vi "Eye_Recorder_v1.0.vi"() -> ()   [LabVIEW 2019]
uses:
  <vilib>/vision/driver/IMAQdx.llb/IMAQdx Acquisition Mode.ctl
  <vilib>/vision/driver/IMAQdx.llb/IMAQdx Buffer Number Mode.ctl
  <vilib>/MakerHub/LINX/Public/Peripherals/Analog/Analog Read N Chans.vi
  <vilib>/MakerHub/LINX/Private/Local IO/LinxAnalogRead.vi
  <vilib>/MakerHub/LINX/Public/Utilities/Check Channel.vi
  <vilib>/MakerHub/LINX/Public/Utilities/Open Serial.vi
  <vilib>/MakerHub/LINX/Private/Utilties/Generate Error.vi
  <vilib>/Utility/file.llb/Write Delimited Spreadsheet (DBL).vi
  <vilib>/vision/driver/NI_Vision_Acquisition_Software.lvlib
  <resource>/objmgr/imaqdx.rc
  <vilib>/vision/NI_Vision_Development_Module.lvlib
  <vilib>/MakerHub/LINX/LMH-LINX.lvlib
panel:
  out "Recording Status":i16[](graph)
  out "Button Status":i16[](graph)
  in  "AI Channel(s)":u8[](array[numeric])=[0, 1]
  out "Experiment Status":i16[](graph)
  in  "AI Threshold":dbl=2.0
  in  "Serial Port":refnum<visa-resource-name>="COM9"
  out "Data Valid":bool
  in  "Centroid Distance Threshold":sgl=5.0
  in  "Initial SD Threshold":sgl=4.0
  in  "SD Threshold Ratio for Stop":sgl=1.2
  in  "SD Threshold Ratio for Start":sgl=1.5
  out "Writing":bool
  in  "Number of Buffered Frames":i32=200
  in  "Smart Record Enable":bool
  out "Actual Frame Rate":dbl=50.04906771344455
  out "Missed Frames":bool
  out "Standard Variation":sgl=5.0659676
  out "Centroid":cluster{"X Centroid":sgl, "Y Centroid":sgl}={"X Centroid"=323.0136, "Y Centroid"=231.01224} {"Y Centroid" format="%.2f"; "X Centroid" format="%.2f"}
  out "Manual ROI":T1={"Global Rectangle"=[0, 0, 639, 479], "Contours"=[{"Contour Type"=0, "ROI Type"=12, "Points"=[0, 0, 639, 479, 0]}]}
  in  "Image Type":T2 items=["Grayscale (U8)", "Grayscale (I16)", "Grayscale (SGL)", "Complex (CSG)", "RGB (U32)", "HSL (U32)", "RGB (U64)", "Grayscale (U16)"]
  in  "Camera Type":enum16{"Basler", "Mako"}(ring)=enum."Mako"
  in  "Folder Path":path=path "C:/Users/VR1/Documents/EyeTrackin/Diego_103019"
  in  "Exposure Time (us)":dbl=15000.0
  out "error out":errorcluster
  in  "Stop":bool
  in  "Byte Order":T3(ring)=enum."little-endian"
  in  "Record?":bool
  in  "File Name (.mtif)":string="test_1"
  out "Size":cluster{"X":i32, "Y":i32}={"X"=640, "Y"=480}
  out "Actual Camera ROI":T4={"Left"=0, "Top"=0, "Right"=639, "Bottom"=479, "Rotation"=0.0} {"Rotation" format="%.2f"; "Left" scale=0.0..1024.0; "Right" scale=0.0..1024.0}
  in  "Set Camera ROI":T4={"Left"=0, "Top"=0, "Right"=639, "Bottom"=479, "Rotation"=0.0} {"Rotation" min=-90.0 max=90.0 step=1.0 format="%.2f"; "Left" scale=0.0..1024.0; "Right" scale=0.0..1024.0}
  out "Raw Image":T5(plugin-control)
  in  "Frame Rate (fps)":dbl=50.0
  in  "Camera Name":refnum<k21>="cam0" caption="IMAQdx Session"
  in  "error in":errorcluster
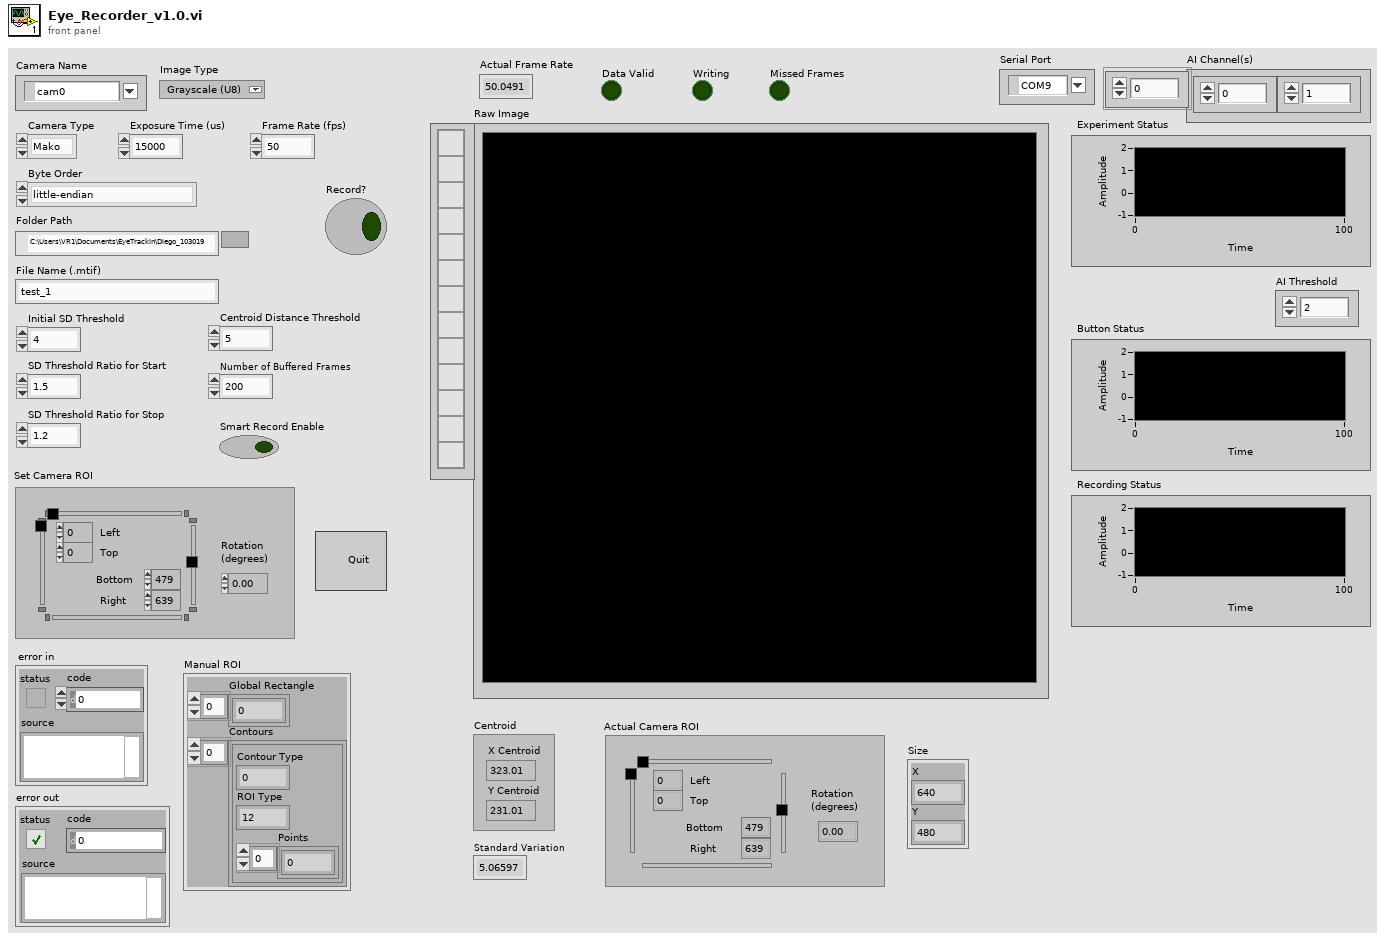
[diagram p1: front panel]
types:
  T1 = cluster{"Global Rectangle":i32[], "Contours":cluster{"Contour Type":u32, "ROI Type":u32, "Points":i32[]}[]}
  T2 = typedef "Image Type" = u32
  T3 = enum16{"big-endian, network order", "native, host order", "little-endian"}
  T4 = typedef "IMAQ Rectangle" = cluster{"Left":i32, "Top":i32, "Right":i32, "Bottom":i32, "Rotation":dbl}
  T5 = typedef "IMAQ Image.ctl" = refnum<image>
  T6 = cluster{"Standard Variation":sgl, "Centroid":cluster{"X Centroid":sgl, "Y Centroid":sgl}}
  T7 = cluster{"ImgDataArray":u8[], "Standard Variation":sgl, "Centroid":cluster{"X Centroid":sgl, "Y Centroid":sgl}}
  T8 = typedef "NI_Vision_Acquisition_Software.lvlib/IMAQdx Acquisition Mode.ctl" = enum32{"One Shot", "Continuous"}
  T9 = typedef "IMAQdx.ctl" = refnum<k21>
  T10 = cluster{"Global Rectangle":i32[], "Contours":cluster{"Contour Type":u32, "Type":u32, "Coordinates":i32[]}[]}
  T11 = typedef "LMH-LINX.lvlib/LINX Ref.ctl" = cluster{"IO":T12, "Interface":T13, "LINX Device Config":T14}
  T12 = typedef "LMH-LINX.lvlib/Platform.ctl" = enum16{"Remote", "Local"}
  T13 = typedef "LMH-LINX.lvlib/Interface.ctl" = enum16{"Serial", "TCP"}
  T14 = typedef "LMH-LINX.lvlib/Device.lvlib/LINX Device Config.ctl" = cluster{"Interface":T13, "COM Port":refnum<visa-resource-name>, "TCP Configuration":T15, "Device Family":u8, "Device ID":u8, "Device Name":string, "TCP Ref":refnum<k5>, "Channels":T16}
  T15 = typedef "LMH-LINX.lvlib/Device.lvlib/TCP Config.ctl" = cluster{"IP Address":string, "Port":u16}
  T16 = typedef "LMH-LINX.lvlib/Channels.ctl" = cluster{"DI":u8[], "DO":u8[], "AI":u8[], "AO":u8[], "PWM":u8[], "QE":u8[], "UART":u8[], "I2C 2":u8[], "SPI":u8[], "CAN":u8[], "Servo":u8[], "AI Ref (V)":dbl, "AI Resolution (Bits)":u8, "AO Ref (V)":dbl, "AO Resolution (Bits)":u8}
  T17 = typedef "NI_Vision_Acquisition_Software.lvlib/IMAQdx Buffer Number Mode.ctl" = enum32{"Next", "Last", "Buffer Number", "Every", "Last New"}
  T18 = cluster{"Mean Value":sgl, "Standard Variation":sgl, "Minimal Value":sgl, "Maximal Value":sgl, "Area (calibrated)":sgl, "Area (pixels)":u32, "%":sgl, "Calibration Valid":bool}
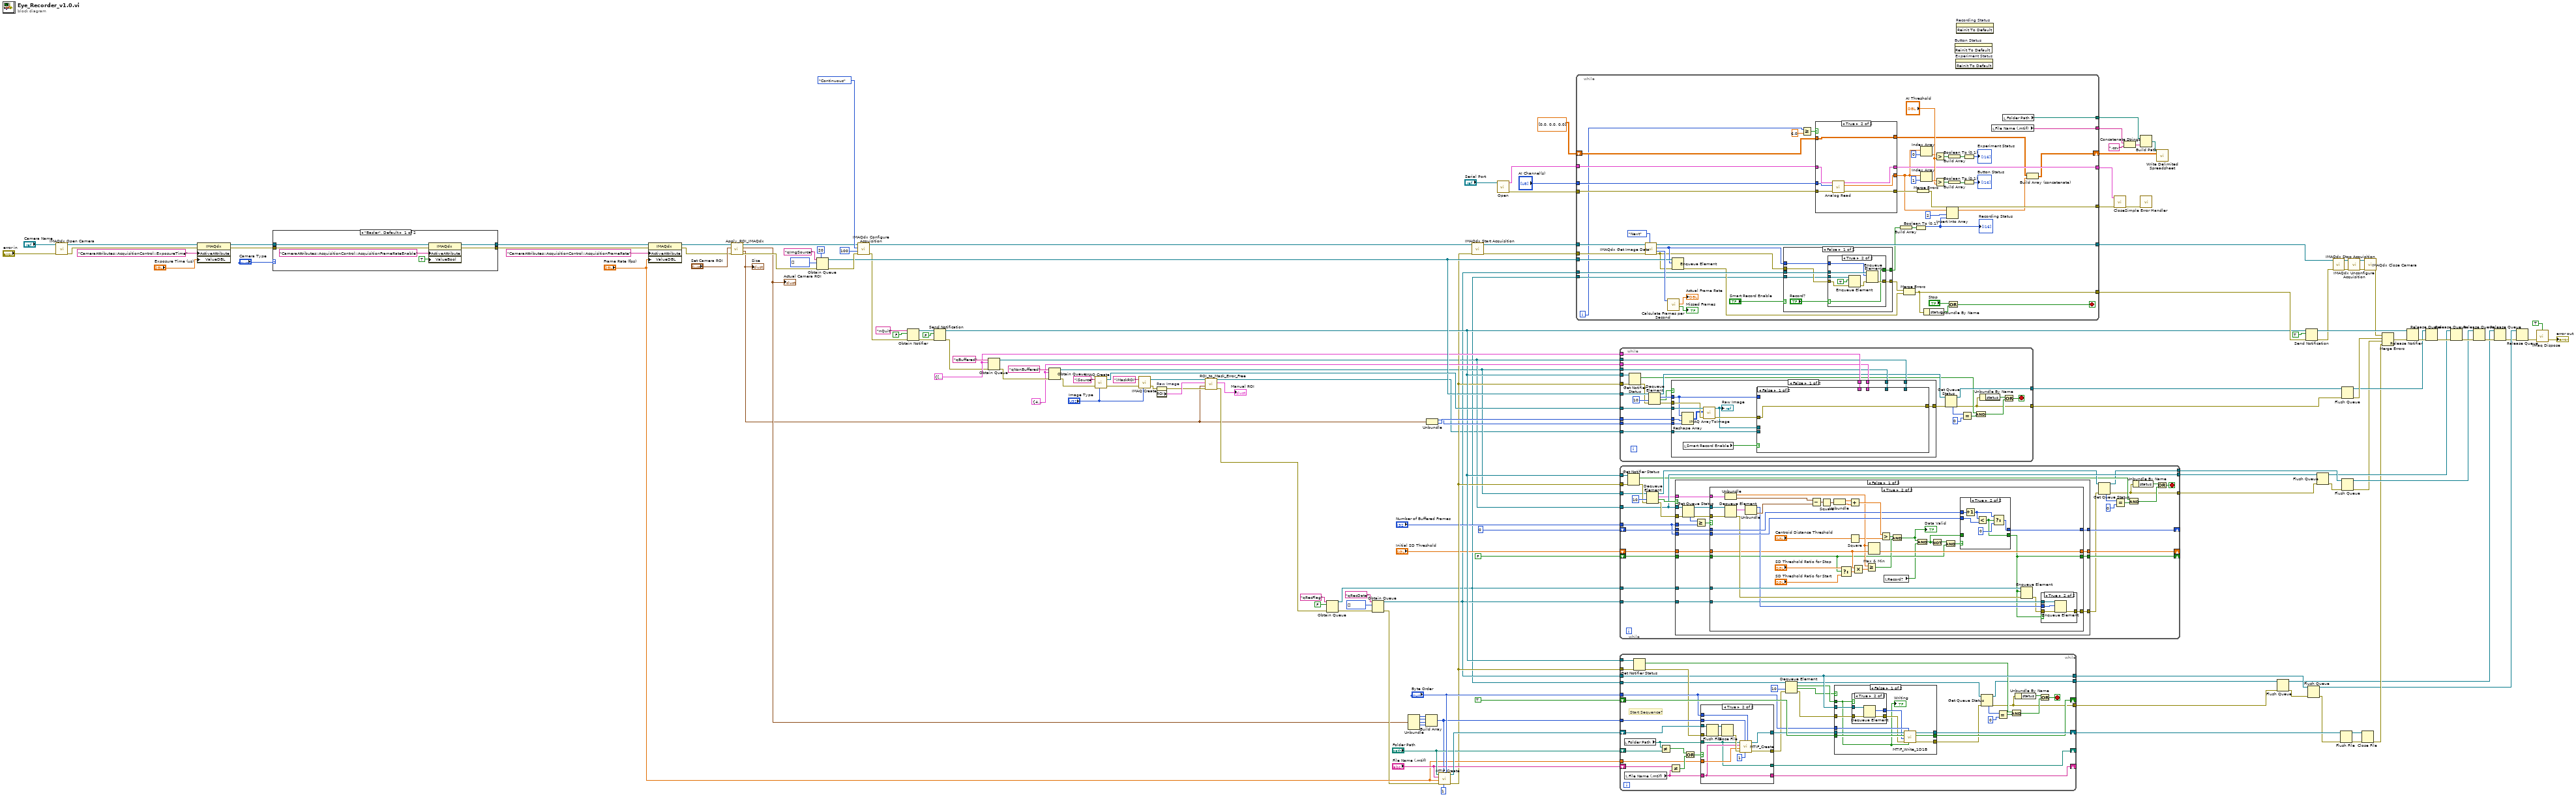
[diagram p0: block diagram]
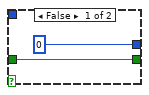
[diagram p4: hidden frame]
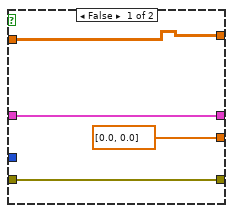
[diagram p6: hidden frame]
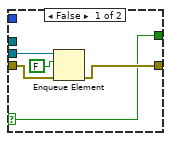
[diagram p7: hidden frame]
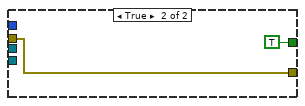
[diagram p8: hidden frame]
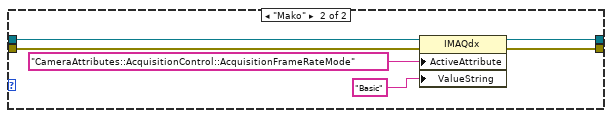
[diagram p9: hidden frame]
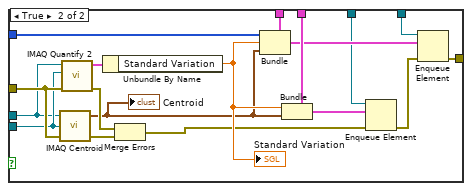
[diagram p10: hidden frame]
diagram:
  w66 = T6 {"Standard Variation"=4836.523, "Centroid"={"X Centroid"=313.66412, "Y Centroid"=260.78278}}
  w67 = T7 {"ImgDataArray"=[], "Standard Variation"=4836.523, "Centroid"={"X Centroid"=313.66412, "Y Centroid"=260.78278}}
  n1 = call <vilib>:"IMAQdx Open Camera.vi"("error in"="error in", "Session In"="Camera Name") -> ("error out"=w96:errorcluster, "Session Out"=w97:T9)  [unwired: 1 in, 7 out]
  n2 = property class="IMAQdx"(reference=w97, error in=w96, "ActiveAttribute"="CameraAttributes::AcquisitionControl::ExposureTime", "ValueDBL"="Exposure Time (us)") -> (reference out=w95:T9, error out=w94:errorcluster)
  n3 = case shown="\"Basler\", Default" "Camera Type" {
    tunnel: w95 -> [w145 w151]
    tunnel: w94 -> [w144 w150]
    tunnel: [w143 w149] -> w93
    tunnel: [w142 w148] -> w92
    frame "Basler", Default {
      n4 = property class="IMAQdx"(reference=w145, error in=w144, "ActiveAttribute"="CameraAttributes::AcquisitionControl::AcquisitionFrameRateEnable", "ValueBool"=TRUE) -> (reference out=w143:T9, error out=w142:errorcluster)
    }
    frame "Mako" {
      n5 = property class="IMAQdx"(reference=w151, error in=w150, "ActiveAttribute"="CameraAttributes::AcquisitionControl::AcquisitionFrameRateMode", "ValueString"="Basic") -> (reference out=w149:T9, error out=w148:errorcluster)
    }
  }
  n6 = property class="IMAQdx"(reference=w93, error in=w92, "ActiveAttribute"="CameraAttributes::AcquisitionControl::AcquisitionFrameRate", "ValueDBL"="Frame Rate (fps)") -> (reference out=w91:T9, error out=w90:errorcluster)
  n7 = call "Apply_ROI_IMAQdx.vi"("error in (no error)"=w90, "ROI"="Set Camera ROI", "Session in"=w91) -> ("error out"=w116:errorcluster, "Size"=w15:cluster{"X":i32, "Y":i32}, "Actual ROI"=w16:T4, "Session out"=w134:T9)  [unwired: 5 in]
  "Actual Camera ROI" <- w16
  "Size" <- w15
  n8 = Obtain Queue(max queue size (-1, unlimited)=20, name (unnamed)="qImgSource", element data type=u8[] [] ("Image Data Array"), error in (no error)=w116) -> (queue out=w76:refnum<queue>, error out=w115:errorcluster)  [unwired: 1 in, 1 out]
  n9 = call <vilib>:"IMAQdx Configure Acquisition.vi"("error in"=w115, "Number of Buffers"=u32 100, "Continuous?"=IMAQdx_Acquisition_Mode."Continuous", "Session In"=w134) -> ("error out"=w64:errorcluster, "Session Out"=w121:T9)  [unwired: 6 in]
  n10 = Obtain Notifier(name (unnamed)="nQuit", notification data type=FALSE ("element"), error in (no error)=w64) -> (notifier out=w111:refnum<notifier>, error out=w110:errorcluster)  [unwired: 1 in, 1 out]
  n11 = Send Notification(notification=FALSE, notifier=w111, error in (no error)=w110) -> (notifier out=w60:refnum<notifier>, error out=w63:errorcluster)
  n12 = Obtain Queue(name (unnamed)="qBuffered", element data type=w67, error in (no error)=w63) -> (queue out=w58:refnum<queue>, error out=w70:errorcluster)  [unwired: 2 in, 1 out]
  n13 = Obtain Queue(name (unnamed)="qNonBuffered", element data type=w66, error in (no error)=w70) -> (queue out=w57:refnum<queue>, error out=w68:errorcluster)  [unwired: 2 in, 1 out]
  n14 = call "IMAQ Create"("Image Name"="iSource", "Image Type"="Image Type", "error in (no error)"=w68) -> ("New Image"=w80:T5, "error out"=w81:errorcluster)  [unwired: 2 in]
  n15 = call "IMAQ Create"("Image Name"="iMaskROI", "Image Type"="Image Type", "error in (no error)"=w81) -> ("New Image"=w22:T5, "error out"=w25:errorcluster)  [unwired: 2 in]
  n16 = property on="Raw Image" class="ImageControl"(error in=w25) -> (error out=w20:errorcluster, "ROI"=w21:T1)  [unwired: 1 in, 1 out]
  n17 = call "ROI_to_Mask_Error_Free.vi"("error in (no error)"=w20, "Image Size"=w15, "ROI in"=w21, "Refnum in"=w22) -> ("error out"=w17:errorcluster, "ROI out"=→"Manual ROI":T10, "Refnum out"=w19:T5)  [unwired: 5 in]
  n18 = Obtain Queue(name (unnamed)="qRecFlag", element data type=FALSE, error in (no error)=w17) -> (queue out=w23:refnum<queue>, error out=w41:errorcluster)  [unwired: 2 in, 1 out]
  n19 = Obtain Queue(name (unnamed)="qRecData", element data type=u8[] [] ("Image Data Array"), error in (no error)=w41) -> (queue out=w24:refnum<queue>, error out=w38:errorcluster)  [unwired: 2 in, 1 out]
  n20 = Unbundle(w16) -> ("Left"=w133:i32, "Top"=w132:i32, "Right"=w131:i32, "Bottom"=w130:i32)  [unwired: 1 out]
  n21 = Build Array(w133, w132, w131, w130) -> (w84:i32[])
  n22 = Unbundle(w15) -> ("X"=w103:i32, "Y"=w104:i32)
  n23 = call "MTIF_Create.vi"("Byte Order"="Byte Order", "Bytes per pixel"=u8 1, "ROI Rectangle"=w84, "error in (no error)"=w38, "Frame Rate (fps)"="Frame Rate (fps)", "File Name (.mtif)"="File Name (.mtif)", "Folder Path"="Folder Path") -> ("error out"=w59:errorcluster, "Byte Stream File out"=w129:refnum<file>)  [unwired: 3 in]
  n24 = call <vilib>:"IMAQdx Start Acquisition.vi"("error in"=w59, "Session In"=w121) -> ("error out"=w77:errorcluster, "Session Out"=w78:T9)  [unwired: 8 in]
  n25 = call-poly <vilib>:"Open.vi"("Serial Port"="Serial Port") -> ("Error Out"=w3:errorcluster, "LINX Resource"=w2:T11)  [unwired: 8 in, 1 out]
  n26 = while {
    tunnel: w78 -> [w200]
    tunnel: w77 -> [w199]
    tunnel: [w196] -> w74
    tunnel: w76 -> [w193]
    tunnel: [w187] -> w73
    tunnel: w24 -> [w190]
    tunnel: w23 -> [w183]
    tunnel: [w168] -> w11
    tunnel: [w167] -> w9
    tunnel: [w166] -> w8
    tunnel: [w165] -> w7
    tunnel: "AI Channel(s)" -> [w164]
    tunnel: w3 -> [w162]
    tunnel: w2 -> [w161]
    shift-right: [w152] -> w1
    shift-left: dbl[][] [[0.0, 0.0, 0.0]] -> [w163]
    i -> [w160]
    stop <- w195 stop-if-true
    n27 = call <vilib>:"IMAQdx Get Image Data.vi"("Buffer Number Mode (Next)"=IMAQdx_Buffer_Number_Mode."Next", "error in"=w199, "Session In"=w200) -> ("error out"=w188:errorcluster, "Buffer Number Out"=w197:u32, "Image Data Array"=w189:u8[], "Session Out"=w196:T9)  [unwired: 5 in]
    n28 = call <vilib>:"Calculate Frames per Second.vi"("Buffer Number"=w197) -> ("Missed Frames"=→"Missed Frames":bool, "Processed Frames/s"=→"Actual Frame Rate":dbl)  [unwired: 8 in, 1 out]
    n29 = Enqueue Element(queue=w193, element=w189, error in (no error)=w188) -> (error out=w186:errorcluster)  [unwired: 1 in, 2 out]
    n30 = case shown="False" "Smart Record Enable" {
      tunnel: w190 -> [w219 _]
      tunnel: w188 -> [w218 w234]
      tunnel: w189 -> [w217 _]
      tunnel: [w216 w234] -> w185
      tunnel: w183 -> [w214 _]
      tunnel: [w213 TRUE] -> w153
      frame False {
        n31 = case shown="True" "Record?" {
          selector: "Record?" -> [w220 w225]
          tunnel: w219 -> [_ w232]
          tunnel: w218 -> [w223 w228]
          tunnel: w217 -> [_ w231]
          tunnel: [w221 w230] -> w216
          tunnel: w214 -> [w224 w229]
          tunnel: [w220 w225] -> w213
          frame False {
            n32 = Enqueue Element(queue=w224, element=FALSE, error in (no error)=w223) -> (error out=w221:errorcluster)  [unwired: 1 in, 2 out]
          }
          frame True {
            n33 = Enqueue Element(queue=w229, element=TRUE, error in (no error)=w228) -> (error out=w226:errorcluster)  [unwired: 1 in, 2 out]
            n34 = Enqueue Element(queue=w232, element=w231, error in (no error)=w226) -> (error out=w230:errorcluster)  [unwired: 1 in, 2 out]
          }
        }
      }
      frame True {
      }
    }
    n35 = Greater Or Equal?(x=w160, y=6.0) -> (x >= y?=w181:bool)
    n36 = case shown="True" w181 {
      tunnel: [w205 w209] -> w165
      tunnel: w162 -> [w204 w212]
      tunnel: w161 -> [w205 w211]
      tunnel: w164 -> [_ w210]
      tunnel: [w204 w208] -> w180
      tunnel: w163 -> [w202 w206]
      tunnel: [w202 w206] -> w155
      tunnel: [dbl[] [0.0, 0.0] ("element") w207] -> w159
      frame False {
      }
      frame True {
        n37 = call-poly <vilib>:"Analog Read.vi"("Error In"=w212, "AI Channel(s)"=w210, "LINX Resource"=w211) -> ("Error Out"=w208:errorcluster, "Voltages"=w207:dbl[], "LINX Resource"=w209:T11)  [unwired: 5 in, 1 out]
      }
    }
    n38 = Build Array(w153) -> (w154:bool[])
    n39 = Merge Errors(w185, w186) -> (w187:errorcluster)
    n40 = Boolean To (0,1)(Boolean=w154) -> (0, 1=w158:i16[])
    "Recording Status" <- w158
    n41 = Merge Errors(w180) -> (w166:errorcluster)
    n42 = Index Array(array=w159, index=0) -> (element=w174:dbl)
    n43 = Index Array(array=w159, index=1) -> (element=w177:dbl)
    n44 = Unbundle By Name(w187) -> ("status"=w194:bool)
    n45 = Greater?(x=w174, y="AI Threshold") -> (0:w182:bool)
    n46 = Greater?(x=w177, y="AI Threshold") -> (0:w178:bool)
    n47 = Insert Into Array(array=w159, index=2, new element=w158) -> (w156:dbl[])
    n48 = Or(x="Stop", y=w194) -> (x .or. y?=w195:bool)
    n49 = Build Array(w182) -> (w172:bool[])
    n50 = Build Array(w178) -> (w179:bool[])
    n51 = Boolean To (0,1)(Boolean=w172) -> (0, 1=→"Experiment Status":i16[])
    n52 = Boolean To (0,1)(Boolean=w179) -> (0, 1=→"Button Status":i16[])
    n53 = local read "File Name (.mtif)"() -> (w168:string)
    n54 = local read "Folder Path"() -> (w167:path)
    n55 = Build Array (concatenate)(w155, w156) -> (w152:dbl[][])
  }
  n56 = while {
    tunnel: w60 -> [w261]
    tunnel: w59 -> [w260]
    tunnel: w76 -> [w258]
    tunnel: w104 -> [w255]
    tunnel: w103 -> [w254]
    tunnel: w80 -> [w253]
    tunnel: [w238] -> w102
    tunnel: w19 -> [w251]
    tunnel: w58 -> [w247]
    tunnel: w57 -> [w246]
    tunnel: w67 -> [w249]
    tunnel: w66 -> [w248]
    tunnel: [w235] -> w37
    stop <- w237 stop-if-true
    n57 = Get Notifier Status(notifier=w261, error in (no error)=w260) -> (current notification=w236:bool, error out=w257:errorcluster)  [unwired: 3 out]
    n58 = Dequeue Element(queue=w258, timeout in ms (-1)=10, error in (no error)=w257) -> (queue out=w239:refnum<queue>, element=w256:u8[], timed out?=w250:bool, error out=w252:errorcluster)
    n59 = case shown="False" w250 {
      tunnel: w256 -> [w263 _]
      tunnel: w255 -> [w276 _]
      tunnel: w254 -> [w275 _]
      tunnel: w253 -> [w274 _]
      tunnel: w252 -> [w273 w296]
      tunnel: w251 -> [w270 _]
      tunnel: [w264 w296] -> w240
      tunnel: w249 -> [w269 _]
      tunnel: w248 -> [w267 _]
      tunnel: w247 -> [w266 _]
      tunnel: w246 -> [w265 _]
      frame False {
        n60 = Reshape Array(w263, w276, w275) -> (w268:u8[][])
        n61 = local read "Smart Record Enable"() -> (w262:bool)
        n62 = call "IMAQ ArrayToImage"("error in (no error)"=w273, "Image Pixels (U8)"=w268, "Image"=w274) -> ("error out"=w272:errorcluster, "Image Out"=w271:T5)  [unwired: 7 in]
        "Raw Image" <- w271
        n63 = case shown="False" w262 {
          tunnel: w272 -> [w277 w293]
          tunnel: w271 -> [_ w278]
          tunnel: w270 -> [_ w292]
          tunnel: w269 -> [_ w290]
          tunnel: w267 -> [_ w289]
          tunnel: w266 -> [_ w286]
          tunnel: w265 -> [_ w283]
          tunnel: [w277 w280] -> w264
          tunnel: w263 -> [_ w279]
          frame False {
          }
          frame True {
            n64 = call "IMAQ Centroid"("error in (no error)"=w293, "Image Mask"=w292, "Image"=w278) -> ("error out"=w291:errorcluster, "Centroid"=w287:cluster{"X Centroid":sgl, "Y Centroid":sgl})  [unwired: 1 in]
            "Centroid" <- w287
            n65 = call "IMAQ Quantify 2"("error in (no error)"=w293, "Image Mask"=w292, "Image"=w278) -> ("error out"=w294:errorcluster, "Global Report"=w295:T18)  [unwired: 6 in, 1 out]
            n66 = Unbundle By Name(w295) -> ("Standard Variation"=w288:sgl)
            "Standard Variation" <- w288
            n67 = Merge Errors(w294, w291) -> (w282:errorcluster)
            n68 = Bundle(cluster=w290, "ImgDataArray"=w279, "Standard Variation"=w288, "Centroid"=w287) -> (w285:T7)
            n69 = Bundle(cluster=w289, "Standard Variation"=w288, "Centroid"=w287) -> (w284:T6)
            n70 = Enqueue Element(queue=w283, element=w284, error in (no error)=w282) -> (error out=w281:errorcluster)  [unwired: 1 in, 2 out]
            n71 = Enqueue Element(queue=w286, element=w285, error in (no error)=w281) -> (error out=w280:errorcluster)  [unwired: 1 in, 2 out]
          }
        }
      }
      frame True {
      }
    }
    n72 = Get Queue Status(queue=w239, error in (no error)=w240) -> (queue out=w238:refnum<queue>, error out=w235:errorcluster, # elements in queue=w245:i32)  [unwired: 1 in, 5 out]
    n73 = Equal?(x=w245, y=0) -> (x = y?=w243:bool)
    n74 = And(x=w236, y=w243) -> (x .and. y?=w241:bool)
    n75 = Unbundle By Name(w235) -> ("status"=w242:bool)
    n76 = Or(x=w242, y=w241) -> (x .or. y?=w237:bool)
  }
  n77 = while {
    tunnel: w60 -> [w324]
    tunnel: w59 -> [w322]
    tunnel: w58 -> [w318]
    tunnel: w57 -> [w321]
    tunnel: "Number of Buffered Frames" -> [w312]
    tunnel: [w297] -> w51
    tunnel: [w318] -> w52
    tunnel: [w298] -> w53
    shift-right: [w314] -> _
    shift-left: "Initial SD Threshold" -> [w316]
    shift-right: [w310] -> _
    shift-left: FALSE -> [w317]
    shift-right: [w311] -> _
    shift-left: 0 ("Number of Buffered Frames") -> [w313]
    tunnel: w23 -> [w308]
    tunnel: w24 -> [w309]
    stop <- w301 stop-if-true
    n78 = Get Notifier Status(notifier=w324, error in (no error)=w322) -> (current notification=w302:bool)  [unwired: 4 out]
    n79 = Dequeue Element(queue=w321, timeout in ms (-1)=10, error in (no error)=w322) -> (queue out=w307:refnum<queue>, element=w315:T6, timed out?=w320:bool, error out=w319:errorcluster)
    n80 = case shown="False" w320 {
      tunnel: w319 -> [w341 w401]
      tunnel: [w337 w401] -> w306
      tunnel: w318 -> [w342 _]
      tunnel: w312 -> [w331 _]
      tunnel: w317 -> [w336 w398]
      tunnel: w316 -> [w335 w400]
      tunnel: w315 -> [w334 _]
      tunnel: [w333 w400] -> w314
      tunnel: w313 -> [w330 w399]
      tunnel: w312 -> [w329 _]
      tunnel: [w328 w399] -> w311
      tunnel: [w327 w398] -> w310
      tunnel: w309 -> [w325 _]
      tunnel: w308 -> [w326 _]
      frame False {
        n81 = Get Queue Status(queue=w342, error in (no error)=w341) -> (queue out=w332:refnum<queue>, error out=w338:errorcluster, # elements in queue=w340:i32)  [unwired: 1 in, 5 out]
        n82 = Greater Or Equal?(x=w340, y=w331) -> (x >= y?=w339:bool)
        n83 = case shown="True" w339 {
          tunnel: [w345 w360] -> w337
          tunnel: w338 -> [w345 w379]
          tunnel: w336 -> [w343 w348]
          tunnel: w335 -> [w346 w359]
          tunnel: w334 -> [_ w382]
          tunnel: [w346 w381] -> w333
          tunnel: w332 -> [_ w380]
          tunnel: w330 -> [w344 w368]
          tunnel: w329 -> [_ w367]
          tunnel: [w344 w366] -> w328
          tunnel: [w343 w354] -> w327
          tunnel: w326 -> [_ w365]
          tunnel: w325 -> [_ w362]
          frame False {
          }
          frame True {
            n84 = Dequeue Element(queue=w380, error in (no error)=w379) -> (element=w378:T7, error out=w364:errorcluster)  [unwired: 1 in, 2 out]
            n85 = Unbundle(w382) -> ("Standard Variation"=w358:sgl, "Centroid"=w377:cluster{"X Centroid":sgl, "Y Centroid":sgl})
            n86 = Unbundle(w378) -> ("ImgDataArray"=w363:u8[], "Centroid"=w376:cluster{"X Centroid":sgl, "Y Centroid":sgl})  [unwired: 1 out]
            n87 = Subtract(x=w377, y=w376) -> (x-y=w375:cluster{"X Centroid":sgl, "Y Centroid":sgl})
            n88 = Square(x=w375) -> (x^2=w374:cluster{"X Centroid":sgl, "Y Centroid":sgl})
            n89 = Unbundle(w374) -> ("X Centroid"=w373:sgl, "Y Centroid"=w372:sgl)
            n90 = Select(t="SD Threshold Ratio for Stop", s=w348, f="SD Threshold Ratio for Start") -> (s? t:f=w384:sgl)
            n91 = Add(x=w373, y=w372) -> (x+y=w371:sgl)
            n92 = Square(x="Centroid Distance Threshold") -> (x^2=w352:sgl)
            n93 = Multiply(x=w359, y=w384) -> (x*y=w383:sgl)
            n94 = Greater Or Equal?(x=w358, y=w383) -> (x >= y?=w370:bool)
            n95 = Max & Min(x=w358, y=w359) -> (min(x,y)=w381:sgl)  [unwired: 1 out]
            n96 = Greater?(x=w371, y=w352) -> (0:w369:bool)
            n97 = local read "Record?"() -> (w347:bool)
            n98 = And(x=w369, y=w370) -> (x .and. y?=w353:bool)
            "Data Valid" <- w353
            n99 = And(x=w353, y=w347) -> (x .and. y?=w357:bool)
            n100 = Not(x=w357) -> (.not. x?=w356:bool)
            n101 = And(x=w356, y=w348) -> (x .and. y?=w355:bool)
            n102 = case shown="True" w355 {
              tunnel: w368 -> [_ w397]
              tunnel: [0 w395] -> w366
              tunnel: w367 -> [_ w393]
              tunnel: w357 -> [w390 _]
              tunnel: [w390 w392] -> w354
              frame False {
              }
              frame True {
                n103 = Increment(x=w397) -> (x+1=w394:i32)
                n104 = Less?(x=w394, y=w393) -> (x < y?=w392:bool)
                n105 = Select(t=w394, s=w392, f=0) -> (s? t:f=w395:i32)
              }
            }
            n106 = Enqueue Element(queue=w365, element=w354, error in (no error)=w364) -> (error out=w361:errorcluster)  [unwired: 1 in, 2 out]
            n107 = case shown="True" w354 {
              tunnel: w363 -> [_ w389]
              tunnel: w362 -> [_ w388]
              tunnel: w361 -> [w385 w387]
              tunnel: [w385 w386] -> w360
              frame False {
              }
              frame True {
                n108 = Enqueue Element(queue=w388, element=w389, error in (no error)=w387) -> (error out=w386:errorcluster)  [unwired: 1 in, 2 out]
              }
            }
          }
        }
      }
      frame True {
      }
    }
    n109 = Get Queue Status(queue=w307, error in (no error)=w306) -> (queue out=w297:refnum<queue>, error out=w298:errorcluster, # elements in queue=w305:i32)  [unwired: 1 in, 5 out]
    n110 = Equal?(x=w305, y=0) -> (x = y?=w303:bool)
    n111 = And(x=w302, y=w303) -> (x .and. y?=w299:bool)
    n112 = Unbundle By Name(w298) -> ("status"=w300:bool)
    n113 = Or(x=w300, y=w299) -> (x .or. y?=w301:bool)
  }
  n114 = while {
    tunnel: "Byte Order" -> [w426]
    shift-right: [w437] -> _
    shift-left: TRUE ("Record?") -> [w438]
    shift-right: [w424] -> _
    shift-left: "Folder Path" -> [w436]
    shift-right: [w425] -> _
    shift-left: "File Name (.mtif)" -> [w430]
    tunnel: w84 -> [w427]
    tunnel: "Frame Rate (fps)" -> [w428]
    shift-right: [w439] -> w124
    shift-left: w129 -> [w432]
    tunnel: w60 -> [w422]
    tunnel: w59 -> [w421]
    tunnel: w23 -> [w419]
    tunnel: w24 -> [w415]
    tunnel: [w415] -> w34
    tunnel: [w403] -> w36
    tunnel: [w402] -> w35
    stop <- w404 stop-if-true
    # "Start Sequence?"
    n115 = local read "Folder Path"() -> (w431:path)
    n116 = local read "File Name (.mtif)"() -> (w429:string)
    n117 = Get Notifier Status(notifier=w422, error in (no error)=w421) -> (current notification=w405:bool, error out=w420:errorcluster)  [unwired: 3 out]
    n118 = Not Equal?(x=w431, y=w436) -> (x != y?=w435:bool)
    n119 = Not Equal?(x=w430, y=w429) -> (x != y?=w434:bool)
    n120 = Or(x=w435, y=w434) -> (x .or. y?=w433:bool)
    n121 = case shown="True" w433 {
      tunnel: w432 -> [w462 w475]
      tunnel: w431 -> [w460 w463]
      tunnel: w429 -> [w459 w464]
      tunnel: w420 -> [w461 w474]
      tunnel: [w462 w467] -> w423
      tunnel: [w461 w466] -> w418
      tunnel: w428 -> [_ w470]
      tunnel: w427 -> [_ w468]
      tunnel: w426 -> [_ w465]
      tunnel: [w459 w464] -> w425
      tunnel: [w460 w463] -> w424
      frame False {
      }
      frame True {
        n122 = Flush File(refnum=w475, error in=w474) -> (refnum out=w473:refnum<file>, error out=w472:errorcluster)
        n123 = Close File(refnum=w473, error in=w472) -> (error out=w471:errorcluster)  [unwired: 1 out]
        n124 = call "MTIF_Create.vi"("Byte Order"=w465, "Bytes per pixel"=u8 1, "ROI Rectangle"=w468, "error in (no error)"=w471, "Frame Rate (fps)"=w470, "File Name (.mtif)"=w464, "Folder Path"=w463) -> ("error out"=w466:errorcluster, "Byte Stream File out"=w467:refnum<file>)  [unwired: 3 in]
      }
    }
    n125 = Dequeue Element(queue=w419, timeout in ms (-1)=10, error in (no error)=w418) -> (queue out=w407:refnum<queue>, element=w414:bool, timed out?=w413:bool, error out=w416:errorcluster)
    n126 = case shown="False" w413 {
      tunnel: [w450 w457] -> w439
      tunnel: w438 -> [w449 w458]
      tunnel: [w448 w458] -> w437
      tunnel: w426 -> [w447 _]
      tunnel: w423 -> [w446 w457]
      tunnel: [w445 w456] -> w406
      tunnel: w416 -> [w444 w456]
      tunnel: w415 -> [w443 _]
      tunnel: w414 -> [w440 _]
      frame False {
        n127 = case shown="True" w440 {
          tunnel: w444 -> [w451 w455]
          tunnel: w443 -> [_ w454]
          tunnel: [w451 w453] -> w442
          tunnel: [_ w452] -> w441
          frame False {
          }
          frame True {
            n128 = Dequeue Element(queue=w454, error in (no error)=w455) -> (element=w452:u8[], error out=w453:errorcluster)  [unwired: 1 in, 2 out]
          }
        }
        n129 = call "MTIF_Write_1D1B.vi"("Record?"=w440, "Byte Order"=w447, "error in (no error)"=w442, "Image Data Array"=w441, "Start Sequence? In"=w449, "Byte Stream File In"=w446) -> ("error out"=w445:errorcluster, "Start Sequence? Out"=w448:bool, "Byte Stream File Out"=w450:refnum<file>)  [unwired: 3 in]
        "Writing" <- w440
      }
      frame True {
      }
    }
    n130 = Get Queue Status(queue=w407, error in (no error)=w406) -> (queue out=w403:refnum<queue>, error out=w402:errorcluster, # elements in queue=w412:i32)  [unwired: 1 in, 5 out]
    n131 = Equal?(x=w412, y=0) -> (x = y?=w410:bool)
    n132 = And(x=w405, y=w410) -> (x .and. y?=w408:bool)
    n133 = Unbundle By Name(w402) -> ("status"=w409:bool)
    n134 = Or(x=w409, y=w408) -> (x .or. y?=w404:bool)
  }
  n135 = invoke on="Button Status" class="WFChart (strict)" method="Reinit To Default"() -> ()  [unwired: 3 in, 3 out]
  n136 = invoke on="Experiment Status" class="WFChart (strict)" method="Reinit To Default"() -> ()  [unwired: 3 in, 3 out]
  n137 = invoke on="Recording Status" class="WFChart (strict)" method="Reinit To Default"() -> ()  [unwired: 3 in, 3 out]
  n138 = call <vilib>:"Close.vi"("Error In"=w8, "LINX Resource"=w7) -> ("Error Out"=w14:errorcluster)  [unwired: 9 in]
  n139 = Concatenate Strings(w11, ".csv" ("string")) -> (w13:string)
  n140 = Build Path(base path=w9, name or relative path=w13) -> (appended path=w12:path)
  n141 = call <vilib>:"Simple Error Handler.vi"("error in (no error)"=w14) -> ()  [unwired: 4 in, 5 out]
  n142 = call-poly <vilib>:"Write Delimited Spreadsheet.vi"("file path (dialog if empty)"=w12, "2D data"=w1) -> ()  [unwired: 12 in, 2 out]
  n143 = Flush Queue(queue=w36, error in (no error)=w35) -> (queue out=w30:refnum<queue>, error out=w33:errorcluster)  [unwired: 1 out]
  n144 = Send Notification(notification=TRUE, notifier=w60, error in (no error)=w73) -> (notifier out=w107:refnum<notifier>, error out=w72:errorcluster)
  n145 = Flush Queue(queue=w34, error in (no error)=w33) -> (queue out=w29:refnum<queue>, error out=w32:errorcluster)  [unwired: 1 out]
  n146 = Flush Queue(queue=w52, error in (no error)=w53) -> (queue out=w48:refnum<queue>, error out=w50:errorcluster)  [unwired: 1 out]
  n147 = call <vilib>:"IMAQdx Stop Acquisition.vi"("error in"=w72, "Session In"=w74) -> ("error out"=w127:errorcluster, "Session Out"=w128:T9)  [unwired: 8 in]
  n148 = Flush File(refnum=w124, error in=w32) -> (refnum out=w123:refnum<file>, error out=w122:errorcluster)
  n149 = Flush Queue(queue=w102, error in (no error)=w37) -> (queue out=w61:refnum<queue>, error out=w62:errorcluster)  [unwired: 1 out]
  n150 = Flush Queue(queue=w51, error in (no error)=w50) -> (queue out=w49:refnum<queue>, error out=w47:errorcluster)  [unwired: 1 out]
  n151 = call <vilib>:"IMAQdx Unconfigure Acquisition.vi"("error in"=w127, "Session In"=w128) -> ("error out"=w126:errorcluster, "Session Out"=w125:T9)  [unwired: 8 in]
  n152 = Close File(refnum=w123, error in=w122) -> (error out=w46:errorcluster)  [unwired: 1 out]
  n153 = call <vilib>:"IMAQdx Close Camera.vi"("error in"=w126, "Session In"=w125) -> ("error out"=w75:errorcluster)  [unwired: 9 out]
  n154 = Merge Errors(w75, w62, w47, w46) -> (w108:errorcluster)
  n155 = Release Notifier(notifier=w107, error in (no error)=w108) -> (error out=w65:errorcluster)  [unwired: 1 in, 2 out]
  n156 = Release Queue(queue=w61, error in (no error)=w65) -> (error out=w55:errorcluster)  [unwired: 1 in, 2 out]
  n157 = Release Queue(queue=w48, error in (no error)=w55) -> (error out=w54:errorcluster)  [unwired: 1 in, 2 out]
  n158 = Release Queue(queue=w49, error in (no error)=w54) -> (error out=w31:errorcluster)  [unwired: 1 in, 2 out]
  n159 = Release Queue(queue=w30, error in (no error)=w31) -> (error out=w28:errorcluster)  [unwired: 1 in, 2 out]
  n160 = Release Queue(queue=w29, error in (no error)=w28) -> (error out=w27:errorcluster)  [unwired: 1 in, 2 out]
  n161 = call "Imaq Dispose"("All Images? (No)"=TRUE, "error in (no error)"=w27) -> ("error out"=→"error out":errorcluster)  [unwired: 1 in, 3 out]
